vi "MPXclearRS232.vi"(1 "MPX COM-Port":refnum<visa-resource-name>="COM5") -> (0 "MPX COM-Port dup":refnum<visa-resource-name>="COM5")   [LabVIEW 2015]
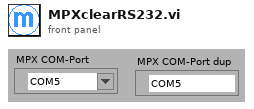
[diagram p1: front panel]
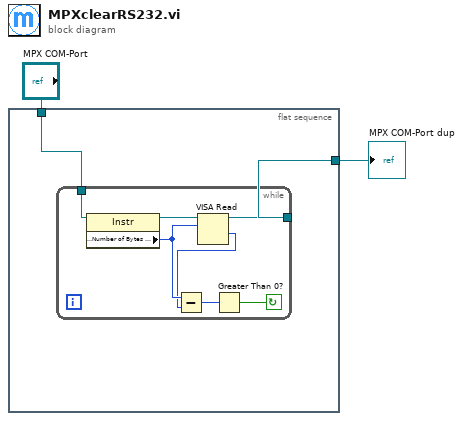
[diagram p0: block diagram]
diagram:
  n1 = flat-sequence {
    tunnel: "MPX COM-Port" -> [w4]
    tunnel: [w3] -> w1
    frame #0 {
      n2 = while {
        tunnel: w4 -> [w7]
        tunnel: [w6] -> w3
        stop <- w10 continue-if-true
        n3 = property class="Instr"(reference=w7) -> (reference out=w11:refnum<visa-resource-name>, "Serial Settings:Number of Bytes at Serial Port"=w9:u32)  [unwired: 1 in, 1 out]
        n4 = VISA Read(VISA resource name=w11, byte count=w9) -> (VISA resource name out=w6:refnum<visa-resource-name>, return count=w8:u32)  [unwired: 1 in, 2 out]
        n5 = Subtract(x=w9, y=w8) -> (x-y=w5:u32)
        n6 = Greater Than 0?(x=w5) -> (x > 0?=w10:bool)
      }
    }
  }
  "MPX COM-Port dup" <- w1
